vi "Begin.vi"(8 "error in":errorcluster) -> (0 "error out":errorcluster)   [LabVIEW 2019]
doc: "Called before other user functions, this VI is expected to open initial I/O refnums, load in file data, and do all program initialization. Notice that the <B>error out</B> terminal is simply used for data flow. Wiring it to other structures or subVIs ensures that this VI runs first."
uses:
  <vilib>/Rock Robotics/WPI/SafetyOutput/WPI_SafetyOutputConfigMenu.ctl
  <vilib>/Rock Robotics/WPI/DriverStation/WPI_DriverStationRobotMode2.ctl
  <vilib>/Rock Robotics/WPI/Joystick/WPI_JoystickDeviceEnum.ctl
  <vilib>/Rock Robotics/SystemInterfaces/DIO/FPGA_DIOChannel.ctl
  <vilib>/Rock Robotics/SystemInterfaces/i2clib/i2c_bus.ctl
  <vilib>/Rock Robotics/WPI/Encoder/WPI_EncoderType.ctl
  Robot Global Data.vi
  <vilib>/Rock Robotics/Network Tables/NT Write String Array.vi
  <vilib>/Rock Robotics/WPI/RobotDrive/WPI_RobotDriveOpen2MotorWithExistingMotors.vi
  <vilib>/Rock Robotics/Network Tables/NT Write Boolean.vi
  <vilib>/Rock Robotics/WPI/Switch/WPI_SwitchOpenLimit.vi
  <vilib>/Rock Robotics/Network Tables/NT Write Number.vi
  <vilib>/Rock Robotics/WPI/Counter/WPI_CounterDigitalInputToDigitalSource.vi
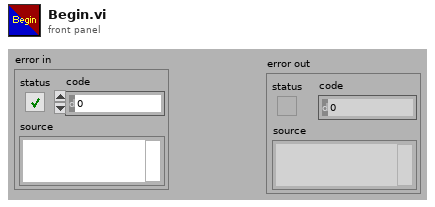
[diagram p1: front panel]
types:
  T1 = typedef "WPI_EncoderType.ctl" = enum16{"1x", "2x", "4x"}
  T2 = typedef "FPGA_DIOChannel.ctl" = enum8{"DIO 0", "DIO 1", "DIO 2", "DIO 3", "DIO 4", "DIO 5", "DIO 6", "DIO 7", "DIO 8", "DIO 9", "DIO MXP 0", "DIO MXP 1", "DIO MXP 2", "DIO MXP 3", "DIO MXP 4", "DIO MXP 5", "DIO MXP 6", "DIO MXP 7", "DIO MXP 8", "DIO MXP 9", "DIO MXP 10", "DIO MXP 11", "DIO MXP 12", "DIO MXP 13", "DIO MXP 14", "DIO MXP 15", "SPI Port CS1", "SPI Port CS2", "SPI Port CS3", "SPI Port MISO", "SPI Port MOSI", "Invalid"}
  T3 = typedef "WPI_JoystickDeviceEnum.ctl" = enum16{"USB 0", "USB 1", "USB 2", "USB 3", "USB 4", "USB 5"}
  T4 = typedef "i2c_bus.ctl" = enum16{"I2C On-Board", "I2C MXP", "Invalid"}
  T5 = typedef "WPI_DriverStationRobotMode2.ctl" = enum16{"Autonomous Disabled", "Autonomous Enabled", "Teleop Disabled", "Teleop Enabled", "Disconnected", "Finish", "Test Disabled", "Test Enabled", "Emergency Stopped"}
  T6 = typedef "WPI_SafetyOutputConfigMenu.ctl" = enum16{"Enable", "Disable"}
  T7 = typedef "WPI_MotorControlDeviceRef.ctl" = cluster{"DeviceStatus":errorcluster, "Type":T8, "PWM":cluster{"PWM Channel":T9, "DeadBand":T10}, "CAN":cluster{"Device Number":u8, "SetOutput VI Ref":variant, "GetOutput VI Ref":variant, "Enable VI Ref":variant, "Disable VI Ref":variant, "Data":variant}, "Invert":bool, "DIO PWM":cluster{"PWM \"Enable\" Channel":T9, "DIOChannel":T2, "PWM Rate":dbl}}
  T8 = typedef "WPI_MotorControlType.ctl" = enum16{"PWM", "CAN", "DIO PWM"}
  T9 = typedef "FPGA_DIOPWMChannel.ctl" = enum8{"PWM 0", "PWM 1", "PWM 2", "PWM 3", "PWM 4", "PWM 5", "PWM 6", "PWM 7", "PWM 8", "PWM 9", "PWM MXP 0", "PWM MXP 1", "PWM MXP 2", "PWM MXP 3", "PWM MXP 4", "PWM MXP 5", "PWM MXP 6", "PWM MXP 7", "PWM MXP 8", "PWM MXP 9", "Invalid"}
  T10 = typedef "WPI_PWMDeadband.ctl" = cluster{"Name":string, "maxPositivePwm":i32, "minPositivePwm":i32, "centerPwm":i32, "maxNegativePwm":i32, "minNegativePwm":i32, "angularRange":u16}
  T11 = typedef "WPI_ServoDeviceRef.ctl" = cluster{"DeviceStatus":errorcluster, "PWM Channel":T9, "DeadBand":T10}
  T12 = typedef "WPI_RobotDriveDevRef.ctl" = cluster{"DevStatus":errorcluster, "Motors[]":T7[], "Square Inputs":bool, "Max Output":dbl}
  T13 = typedef "WPI_JoystickDevRef.ctl" = cluster{"Device":T3}
  T14 = typedef "WPI_SwitchDevRef.ctl" = cluster{"DevStatus":errorcluster, "DIO Channel":T2, "CntIndex":T15, "Normally Closed":bool}
  T15 = typedef "FPGA_CounterCtrSystemIndex.ctl" = enum8{"Ctr 0", "Ctr 1", "Ctr 2", "Ctr 3", "Ctr 4", "Ctr 5", "Ctr 6", "Ctr 7", "Invalid"}
  T16 = typedef "Color Sensor V3 DevRef.ctl" = cluster{"I2CDevRef":T17}
  T17 = typedef "WPI_I2CDevRef.ctl" = cluster{"DevStatus":errorcluster, "Device Address":u8, "Handle":i32, "I2C Bus":T4}
  T18 = typedef "WPI_DigitalInputDevRef.ctl" = cluster{"DevStatus":errorcluster, "DIO Channel":T2}
  T19 = typedef "FPGA_CounterEncoderSourceConvertionLVSourceType.ctl" = cluster{"DevStatus":errorcluster, "AnalogTriggerMode?":bool, "DigitalMode":cluster{"DIO Channel":T20}, "AnalogTriggerMode":cluster{"AnalogTriggerIndex":T21, "OutputType":T22}}
  T20 = typedef "FPGA_DIODigitalSourceChannel.ctl" = enum8{"DIO 0", "DIO 1", "DIO 2", "DIO 3", "DIO 4", "DIO 5", "DIO 6", "DIO 7", "DIO 8", "DIO 9", "DIO MXP 0", "DIO MXP 1", "DIO MXP 2", "DIO MXP 3", "DIO MXP 4", "DIO MXP 5", "DIO MXP 6", "DIO MXP 7", "DIO MXP 8", "DIO MXP 9", "DIO MXP 10", "DIO MXP 11", "DIO MXP 12", "DIO MXP 13", "DIO MXP 14", "DIO MXP 15", "SPI Port CS1", "SPI Port CS2", "SPI Port CS3", "SPI Port MISO", "SPI Port MOSI", "Disabled"}
  T21 = typedef "FPGA_AnalogTriggerIndex.ctl" = enum8{"Trig 0", "Trig 1", "Trig 2", "Trig 3", "Trig 4", "Trig 5", "Trig 6", "Trig 7", "Invalid"}
  T22 = typedef "FPGA_AnalogTriggerOutType.ctl" = enum16{"InWindow", "TriggerState", "Rising", "Falling"}
  T23 = typedef "WPI_EncoderDevRef.ctl" = cluster{"DevStatus":errorcluster, "EncoderIndex":T24, "CounterIndex":T15, "DistancePerCount":dbl, "Decoding Type":T1}
  T24 = typedef "FPGA_EncoderIdx.ctl" = enum8{"Enc 0", "Enc 1", "Enc 2", "Enc 3", "Enc 4", "Enc 5", "Enc 6", "Enc 7", "Invalid"}
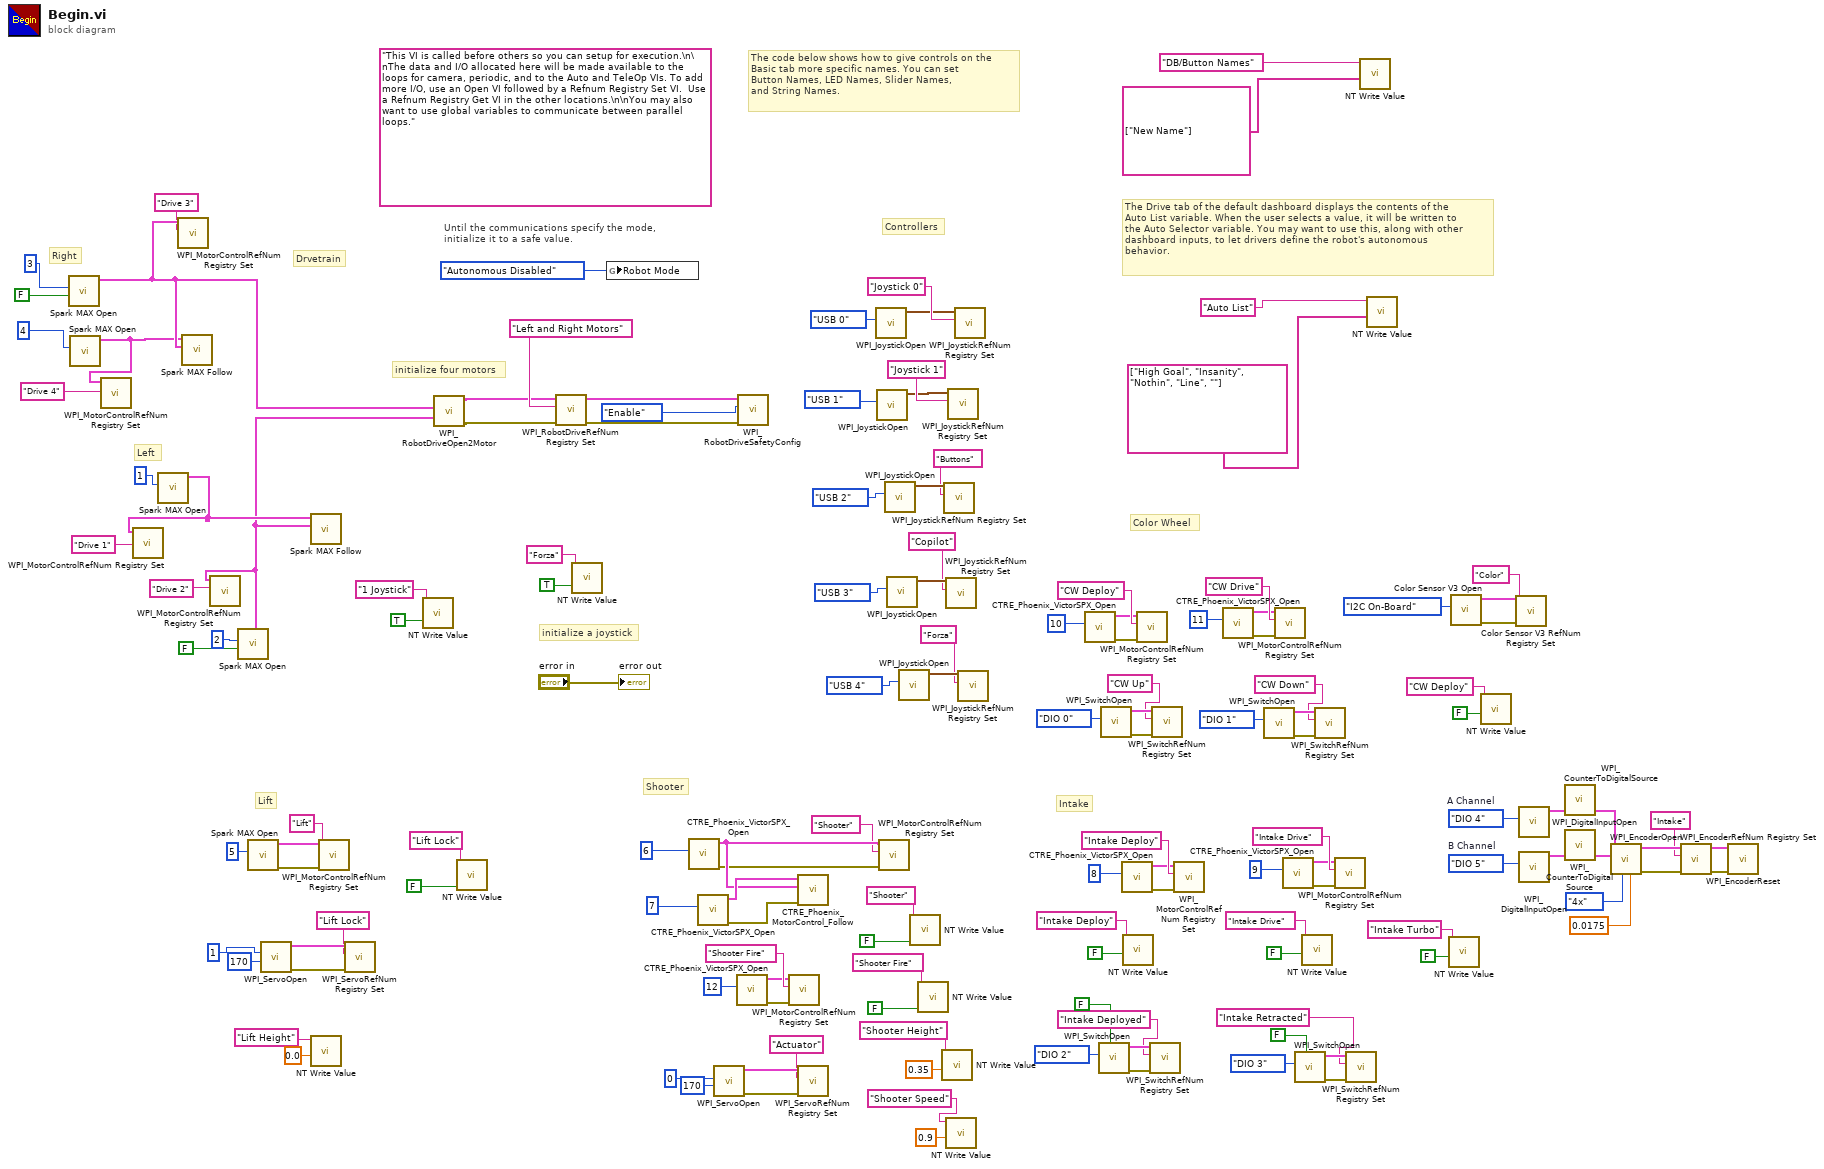
[diagram p0: block diagram]
diagram:
  w18 = FPGA_DIOChannel."DIO 5"  # B Channel
  w17 = FPGA_DIOChannel."DIO 4"  # A Channel
  (unwired) "This VI is called before others so you can setup for execution.\n\nThe data and I/O allocated here will be made available to the loops for camera, periodic, and to the Auto and TeleOp VIs. To add more I/O, use an Open VI followed by a Refnum Registry Set VI.  Use a Refnum Registry Get VI in the other locations.\n\nYou may also want to use global variables to communicate between parallel loops."
  # "Drvetrain"
  # "Controllers"
  # "Lift"
  # "Shooter"
  # "Color Wheel"
  # "Intake"
  # "Right"
  # "Left"
  # "The Drive tab of the default dashboard displays the contents of the\nAuto List variable. When the user selects a value, it will be written to\nthe Auto Selector variable. You may want to use this, along with other\ndashboard inputs, to let drivers define the robot's autonomous\nbehavior."
  # "The code below shows how to give controls on the\nBasic tab more specific names. You can set\nButton Names, LED Names, Slider Names,\nand String Names."
  # "initialize a joystick"
  # "Until the communications specify the mode,\ninitialize it to a safe value."
  # "initialize four motors"
  n1 = call <vilib>:"Spark MAX Open.vi"("Invert"=FALSE ("RightMotorInverted"), "Device Number"=3) -> ("MotorControlDeviceRef"=w119:T7)  [unwired: 8 in, 1 out]
  n2 = call <vilib>:"Spark MAX Open.vi"("Device Number"=4) -> ("MotorControlDeviceRef"=w118:T7)  [unwired: 9 in, 1 out]
  n3 = call <vilib>:"WPI_MotorControlRefNum Registry Set.vi"("refnum name"="Drive 4", "MotorControlDevRef"=w118) -> ()  [unwired: 8 in, 2 out]
  n4 = call <vilib>:"Spark MAX Open.vi"("Device Number"=1) -> ("MotorControlDeviceRef"=w117:T7)  [unwired: 9 in, 1 out]
  n5 = call <vilib>:"WPI_MotorControlRefNum Registry Set.vi"("refnum name"="Drive 1", "MotorControlDevRef"=w117) -> ()  [unwired: 8 in, 2 out]
  n6 = call <vilib>:"WPI_MotorControlRefNum Registry Set.vi"("refnum name"="Drive 3", "MotorControlDevRef"=w119) -> ()  [unwired: 8 in, 2 out]
  n7 = call <vilib>:"Spark MAX Follow.vi"("Master Controller"=w119, "MotorControlDeviceRef"=w118) -> ()  [unwired: 8 in, 2 out]
  n8 = call <vilib>:"Spark MAX Open.vi"("Invert"=FALSE ("LeftMotorInverted"), "Device Number"=2) -> ("MotorControlDeviceRef"=w116:T7)  [unwired: 8 in, 1 out]
  n9 = call <vilib>:"WPI_MotorControlRefNum Registry Set.vi"("refnum name"="Drive 2", "MotorControlDevRef"=w116) -> ()  [unwired: 8 in, 2 out]
  n10 = call <vilib>:"Spark MAX Open.vi"("Device Number"=u8 5) -> ("error out"=w73:errorcluster, "MotorControlDeviceRef"=w72:T7)  [unwired: 9 in]
  n11 = call <vilib>:"WPI_ServoOpen.vi"("Angular Range"=u16 170, "PWM Channel"=1) -> ("error out"=w50:errorcluster, "ServoDeviceRef"=w52:T11)  [unwired: 8 in]
  n12 = call <vilib>:"Spark MAX Follow.vi"("Master Controller"=w116, "MotorControlDeviceRef"=w117) -> ()  [unwired: 8 in, 2 out]
  n13 = call-poly <vilib>:"NT Write Value.vi"("Numeric"=0.0, "Name"="Lift Height") -> ()  [unwired: 9 in, 1 out]
  n14 = call <vilib>:"WPI_MotorControlRefNum Registry Set.vi"("error in (no error)"=w73, "refnum name"="Lift", "MotorControlDevRef"=w72) -> ()  [unwired: 7 in, 2 out]
  n15 = call <vilib>:"WPI_ServoRefNum Registry Set.vi"("error in (no error)"=w50, "refnum name"="Lift Lock", "ServoDeviceRef"=w52) -> ()  [unwired: 7 in, 2 out]
  n16 = call-poly <vilib>:"NT Write Value.vi"("Boolean"=TRUE, "Name"="1 Joystick") -> ()  [unwired: 9 in, 1 out]
  n17 = call-poly <vilib>:"WPI_RobotDriveOpen2Motor.vi"("Right Motor Dev Ref"=w119, "Left Motor Dev Ref"=w116) -> ("error out"=w68:errorcluster, "RobotDriveDevRef"=w122:T12)  [unwired: 8 in]
  n18 = call-poly <vilib>:"NT Write Value.vi"("Boolean"=FALSE, "Name"="Lift Lock") -> ()  [unwired: 9 in, 1 out]
  n19 = call <vilib>:"WPI_RobotDriveRefNum Registry Set.vi"("error in (no error)"=w68, "refnum name"="Left and Right Motors", "RobotDriveDevRef"=w122) -> ("error out"=w69:errorcluster, "RobotDriveDevRef"=w140:T12)  [unwired: 1 in, 6 out]
  n20 = call-poly <vilib>:"NT Write Value.vi"("Boolean"=TRUE, "Name"="Forza") -> ()  [unwired: 9 in, 1 out]
  n21 = global write "Robot Global Data.vi" "Robot Mode"(WPI_DriverStationRobotMode2."Autonomous Disabled" ("Robot Mode")) -> ()
  n22 = call <vilib>:"CTRE_Phoenix_VictorSPX_Open.vi"("Device Number"=6) -> ("error out"=w66:errorcluster, "CAN Talon SRX Ref"=w105:T7)  [unwired: 9 in]
  n23 = call <vilib>:"CTRE_Phoenix_VictorSPX_Open.vi"("Device Number"=7) -> ("error out"=w67:errorcluster, "CAN Talon SRX Ref"=w111:T7)  [unwired: 9 in]
  n24 = call <vilib>:"WPI_ServoOpen.vi"("Angular Range"=u16 170, "PWM Channel"=0) -> ("error out"=w65:errorcluster, "ServoDeviceRef"=w108:T11)  [unwired: 8 in]
  n25 = call <vilib>:"CTRE_Phoenix_VictorSPX_Open.vi"("Device Number"=12) -> ("error out"=w46:errorcluster, "CAN Talon SRX Ref"=w47:T7)  [unwired: 9 in]
  n26 = call <vilib>:"WPI_RobotDriveSafetyConfig.vi"("error in (no error)"=w69, "mode"=WPI_SafetyOutputConfigMenu."Enable", "RobotDriveDevRef"=w140) -> ()  [unwired: 7 in, 2 out]
  n27 = call <vilib>:"WPI_MotorControlRefNum Registry Set.vi"("error in (no error)"=w46, "refnum name"="Shooter Fire", "MotorControlDevRef"=w47) -> ()  [unwired: 7 in, 2 out]
  n28 = call <vilib>:"CTRE_Phoenix_MotorControl_Follow.vi"("error in (no error)"=w67, "Master Controller to Follow"=w105, "PhoenixMotorControlDevRef"=w111) -> ()  [unwired: 7 in, 2 out]
  n29 = call <vilib>:"WPI_ServoRefNum Registry Set.vi"("error in (no error)"=w65, "refnum name"="Actuator", "ServoDeviceRef"=w108) -> ()  [unwired: 7 in, 2 out]
  n30 = call <vilib>:"WPI_JoystickOpen.vi"("JoystickDevice"=WPI_JoystickDeviceEnum."USB 0") -> ("JoystickDevRef"=w136:T13)  [unwired: 10 in]
  n31 = call <vilib>:"WPI_JoystickOpen.vi"("JoystickDevice"=WPI_JoystickDeviceEnum."USB 1") -> ("JoystickDevRef"=w56:T13)  [unwired: 10 in]
  n32 = call <vilib>:"WPI_MotorControlRefNum Registry Set.vi"("error in (no error)"=w66, "refnum name"="Shooter", "MotorControlDevRef"=w105) -> ()  [unwired: 7 in, 2 out]
  n33 = call <vilib>:"WPI_JoystickOpen.vi"("JoystickDevice"=WPI_JoystickDeviceEnum."USB 2") -> ("JoystickDevRef"=w59:T13)  [unwired: 10 in]
  n34 = call <vilib>:"WPI_JoystickOpen.vi"("JoystickDevice"=WPI_JoystickDeviceEnum."USB 3") -> ("JoystickDevRef"=w128:T13)  [unwired: 10 in]
  n35 = call <vilib>:"WPI_JoystickOpen.vi"("JoystickDevice"=WPI_JoystickDeviceEnum."USB 4") -> ("JoystickDevRef"=w42:T13)  [unwired: 10 in]
  n36 = call-poly <vilib>:"NT Write Value.vi"("Boolean"=FALSE, "Name"="Shooter") -> ()  [unwired: 9 in, 1 out]
  n37 = call-poly <vilib>:"NT Write Value.vi"("Boolean"=FALSE, "Name"="Shooter Fire") -> ()  [unwired: 9 in, 1 out]
  n38 = call-poly <vilib>:"NT Write Value.vi"("Numeric"=0.35, "Name"="Shooter Height") -> ()  [unwired: 9 in, 1 out]
  n39 = call <vilib>:"WPI_JoystickRefNum Registry Set.vi"("refnum name"="Buttons", "JoystickDevRef"=w59) -> ()  [unwired: 8 in, 2 out]
  n40 = call <vilib>:"WPI_JoystickRefNum Registry Set.vi"("refnum name"="Copilot", "JoystickDevRef"=w128) -> ()  [unwired: 8 in, 2 out]
  n41 = call-poly <vilib>:"NT Write Value.vi"("Numeric"=0.9, "Name"="Shooter Speed") -> ()  [unwired: 9 in, 1 out]
  n42 = call <vilib>:"WPI_JoystickRefNum Registry Set.vi"("refnum name"="Joystick 1", "JoystickDevRef"=w56) -> ()  [unwired: 8 in, 2 out]
  n43 = call <vilib>:"WPI_JoystickRefNum Registry Set.vi"("refnum name"="Joystick 0", "JoystickDevRef"=w136) -> ()  [unwired: 8 in, 2 out]
  n44 = call <vilib>:"WPI_JoystickRefNum Registry Set.vi"("refnum name"="Forza", "JoystickDevRef"=w42) -> ()  [unwired: 8 in, 2 out]
  n45 = call <vilib>:"CTRE_Phoenix_VictorSPX_Open.vi"("Device Number"=10) -> ("error out"=w87:errorcluster, "CAN Talon SRX Ref"=w88:T7)  [unwired: 9 in]
  n46 = call-poly <vilib>:"WPI_SwitchOpen.vi"("Normally Closed"=FALSE, "DIO Channel"=FPGA_DIOChannel."DIO 2") -> ("error out"=w39:errorcluster, "SwitchDevRef"=w38:T14)  [unwired: 8 in]
  n47 = call-poly <vilib>:"WPI_SwitchOpen.vi"("DIO Channel"=FPGA_DIOChannel."DIO 0") -> ("error out"=w81:errorcluster, "SwitchDevRef"=w80:T14)  [unwired: 9 in]
  n48 = call <vilib>:"CTRE_Phoenix_VictorSPX_Open.vi"("Device Number"=8) -> ("error out"=w97:errorcluster, "CAN Talon SRX Ref"=w98:T7)  [unwired: 9 in]
  n49 = call-poly <vilib>:"NT Write Value.vi"("Boolean"=FALSE, "Name"="Intake Deploy") -> ()  [unwired: 9 in, 1 out]
  n50 = call <vilib>:"WPI_MotorControlRefNum Registry Set.vi"("error in (no error)"=w87, "refnum name"="CW Deploy", "MotorControlDevRef"=w88) -> ()  [unwired: 7 in, 2 out]
  n51 = call <vilib>:"WPI_SwitchRefNum Registry Set.vi"("error in (no error)"=w39, "refnum name"="Intake Deployed", "SwitchDevRef"=w38) -> ()  [unwired: 7 in, 2 out]
  n52 = call <vilib>:"WPI_SwitchRefNum Registry Set.vi"("error in (no error)"=w81, "refnum name"="CW Up", "SwitchDevRef"=w80) -> ()  [unwired: 7 in, 2 out]
  n53 = call <vilib>:"WPI_MotorControlRefNum Registry Set.vi"("error in (no error)"=w97, "refnum name"="Intake Deploy", "MotorControlDevRef"=w98) -> ()  [unwired: 7 in, 2 out]
  n54 = call <vilib>:"CTRE_Phoenix_VictorSPX_Open.vi"("Device Number"=11) -> ("error out"=w83:errorcluster, "CAN Talon SRX Ref"=w84:T7)  [unwired: 9 in]
  n55 = call-poly <vilib>:"WPI_SwitchOpen.vi"("DIO Channel"=FPGA_DIOChannel."DIO 1") -> ("error out"=w78:errorcluster, "SwitchDevRef"=w77:T14)  [unwired: 9 in]
  n56 = call <vilib>:"WPI_MotorControlRefNum Registry Set.vi"("error in (no error)"=w83, "refnum name"="CW Drive", "MotorControlDevRef"=w84) -> ()  [unwired: 7 in, 2 out]
  n57 = call <vilib>:"CTRE_Phoenix_VictorSPX_Open.vi"("Device Number"=9) -> ("error out"=w91:errorcluster, "CAN Talon SRX Ref"=w92:T7)  [unwired: 9 in]
  n58 = call-poly <vilib>:"WPI_SwitchOpen.vi"("Normally Closed"=FALSE, "DIO Channel"=FPGA_DIOChannel."DIO 3") -> ("error out"=w35:errorcluster, "SwitchDevRef"=w34:T14)  [unwired: 8 in]
  n59 = call-poly <vilib>:"NT Write Value.vi"("Boolean"=FALSE, "Name"="Intake Drive") -> ()  [unwired: 9 in, 1 out]
  n60 = call <vilib>:"WPI_SwitchRefNum Registry Set.vi"("error in (no error)"=w78, "refnum name"="CW Down", "SwitchDevRef"=w77) -> ()  [unwired: 7 in, 2 out]
  n61 = call <vilib>:"WPI_MotorControlRefNum Registry Set.vi"("error in (no error)"=w91, "refnum name"="Intake Drive", "MotorControlDevRef"=w92) -> ()  [unwired: 7 in, 2 out]
  n62 = call <vilib>:"WPI_SwitchRefNum Registry Set.vi"("error in (no error)"=w35, "refnum name"="Intake Retracted", "SwitchDevRef"=w34) -> ()  [unwired: 7 in, 2 out]
  n63 = call-poly <vilib>:"NT Write Value.vi"("String Array"=string[] ["New Name"], "Name"="DB/Button Names") -> ()  [unwired: 9 in, 1 out]
  n64 = call-poly <vilib>:"NT Write Value.vi"("String Array"=string[] ["High Goal", "Insanity", "Nothin", "Line", ""], "Name"="Auto List") -> ()  [unwired: 9 in, 1 out]
  n65 = call-poly <vilib>:"NT Write Value.vi"("Boolean"=FALSE, "Name"="Intake Turbo") -> ()  [unwired: 9 in, 1 out]
  n66 = call <vilib>:"Color Sensor V3 Open.vi"("I2C Bus"=i2c_bus."I2C On-Board") -> ("error out"=w103:errorcluster, "ColorSensorDevRef"=w102:T16)  [unwired: 9 in]
  n67 = call-poly <vilib>:"NT Write Value.vi"("Boolean"=FALSE, "Name"="CW Deploy") -> ()  [unwired: 9 in, 1 out]
  n68 = call <vilib>:"Color Sensor V3 RefNum Registry Set.vi"("error in (no error)"=w103, "refnum name"="Color", "ColorSensorDevRef"=w102) -> ()  [unwired: 7 in, 2 out]
  n69 = call <vilib>:"WPI_DigitalInputOpen.vi"("DIO Channel"=w17) -> ("DigitalInputDevRef"=w14:T18)  [unwired: 1 in, 9 out]
  n70 = call <vilib>:"WPI_DigitalInputOpen.vi"("DIO Channel"=w18) -> ("DigitalInputDevRef"=w15:T18)  [unwired: 1 in, 9 out]
  n71 = call-poly <vilib>:"WPI_CounterToDigitalSource.vi"("DigitalInputDevRef"=w14) -> ("Digital Source"=w13:T19)  [unwired: 6 out]
  n72 = call-poly <vilib>:"WPI_CounterToDigitalSource.vi"("DigitalInputDevRef"=w15) -> ("Digital Source"=w16:T19)  [unwired: 6 out]
  n73 = call <vilib>:"WPI_EncoderOpen.vi"("DistancePerCount"=0.0175, "Decoding Type"=WPI_EncoderType."4x", "BSource"=w16, "ASource"=w13) -> ("error out"=w12:errorcluster, "EncoderDevRef"=w11:T23)  [unwired: 4 in, 2 out]
  n74 = call <vilib>:"WPI_EncoderRefNum Registry Set.vi"("error in (no error)"=w12, "refnum name"="Intake", "EncoderDevRef"=w11) -> ("error out"=w9:errorcluster, "EncoderDevRef"=w8:T23)  [unwired: 7 in]
  n75 = call <vilib>:"WPI_EncoderReset.vi"("error in (no error)"=w9, "EncoderDevRef"=w8) -> ()  [unwired: 8 in, 2 out]
  "error out" <- "error in"
